vi "Gen Cycle.vi"(7 "Real Time State":T1, 9 "Gen East":T2 {"TotalFuel(L)" format="%.2f"; "FuelRate(L/H)" format="%.2f"; "ApparentPower(VA)" format="%.2f"; "BattVoltage(V)" format="%.2f"; "Freq(Hz)" format="%.2f"; "RunHours(hr)" format="%.2f"; "PowerFactor" format="%.2f"; "ReactivePower(VAR)" format="%.2f"; "ActivePower(W)" format="%.2f"}, 10 "Gen West":T2 {"TotalFuel(L)" format="%.2f"; "FuelRate(L/H)" format="%.2f"; "ApparentPower(VA)" format="%.2f"; "BattVoltage(V)" format="%.2f"; "Freq(Hz)" format="%.2f"; "RunHours(hr)" format="%.2f"; "PowerFactor" format="%.2f"; "ReactivePower(VAR)" format="%.2f"; "ActivePower(W)" format="%.2f"}, 11 "Generator ON":bool=TRUE) -> (1 "Gen Active":T2 {"TotalFuel(L)" format="%.2f"; "FuelRate(L/H)" format="%.2f"; "ApparentPower(VA)" format="%.2f"; "BattVoltage(V)" format="%.2f"; "Freq(Hz)" format="%.2f"; "RunHours(hr)" format="%.2f"; "PowerFactor" format="%.2f"; "ReactivePower(VAR)" format="%.2f"; "ActivePower(W)" format="%.2f"}, 2 "Generator ON East":bool=TRUE, 3 "Generator ON West":bool=TRUE)   [LabVIEW 2014]
uses:
  Controls/Gen Data.ctl
  Controls/RT State.ctl
panel:
  out "Gen West Not Ready":bool=TRUE
  out "Gen East Not Ready":bool=TRUE
  in  "Hour":i32=12
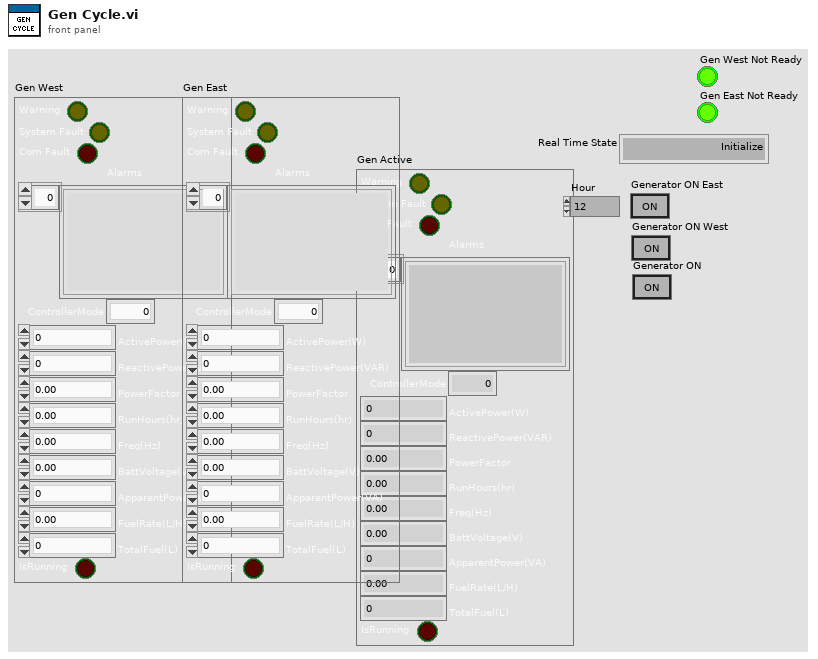
[diagram p1: front panel]
types:
  T1 = typedef "RT State.ctl" = enum16{"Initialize", "Ready", "Startup 1 - Start Genset", "Startup 2 - Start Inverter", "Startup 3 - Battery Match", "SpotGen - Start", "SpotGen - Charge", "SpotGen - Desync", "SpotGen - Discharge", "SpotGen - Sync", "Shutdown", "INVALID STATE"}
  T2 = typedef "Gen Data.ctl" = cluster{"Warning":bool, "System Fault":bool, "Com Fault":bool, "Alarms":string[], "ControllerMode":u16, "ActivePower(W)":i32, "ReactivePower(VAR)":i32, "PowerFactor":dbl, "RunHours(hr)":dbl, "Freq(Hz)":dbl, "BattVoltage(V)":dbl, "ApparentPower(VA)":i32, "FuelRate(L/H)":dbl, "TotalFuel(L)":u32, "IsRunning":bool}
  T3 = typedef "LVDateTimeRec.ctl" = cluster{"fractional second":dbl, "second":i32, "minute":i32, "hour":i32, "day of month":i32, "month":i32, "year":i32, "day of week":i32, "day of year":i32, "DST":i32}
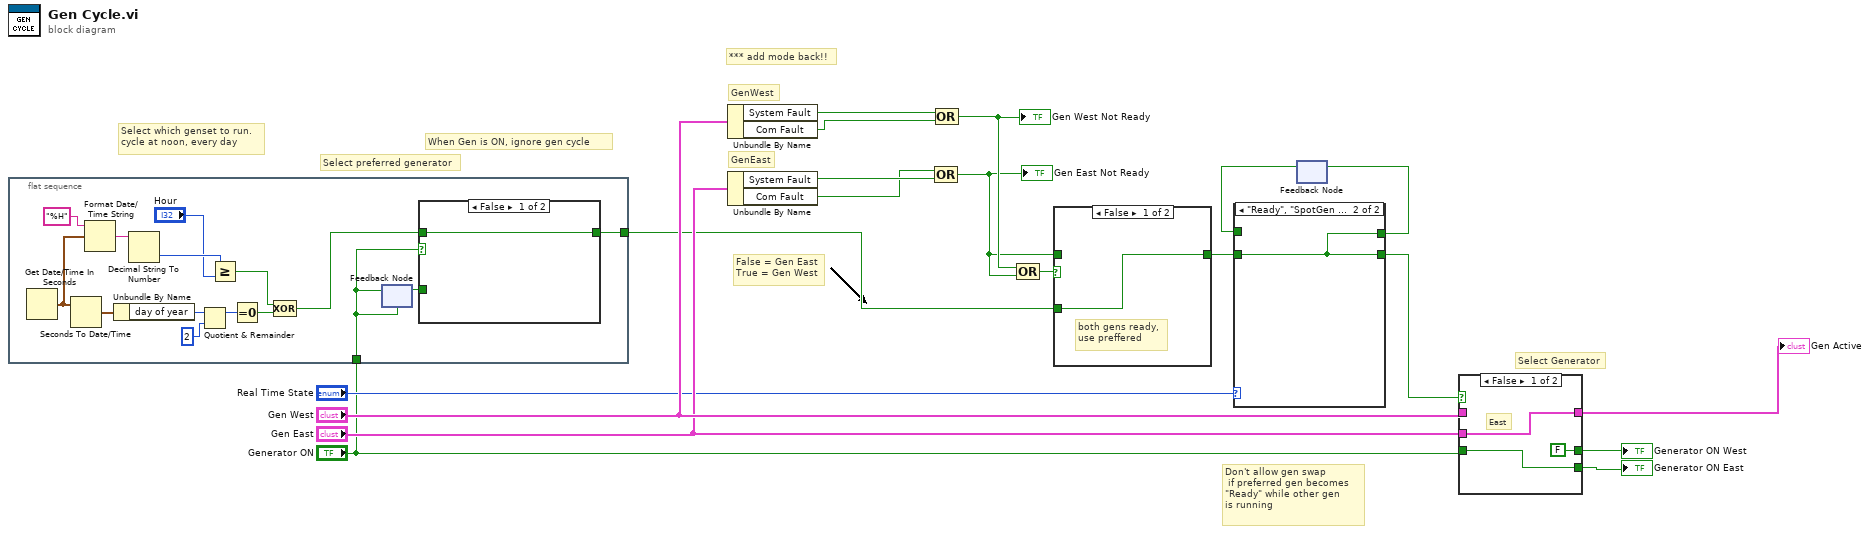
[diagram p0: block diagram]
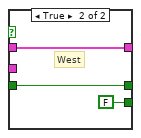
[diagram p4: hidden frame]
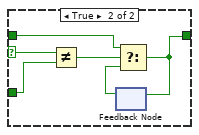
[diagram p5: hidden frame]
diagram:
  # "*** add mode back!!"
  # "GenEast"
  # "GenWest"
  # "Select preferred generator"
  # "Don't allow gen swap \n if preferred gen becomes \n\"Ready\" while other gen \nis running"
  # "Select Generator"
  # "False = Gen East\nTrue = Gen West"
  # "When Gen is ON, ignore gen cycle"
  # "Select which genset to run.\ncycle at noon, every day"
  n1 = flat-sequence {
    tunnel: "Generator ON" -> [w21]
    tunnel: [w20] -> w14
    frame #0 {
      n2 = Get Date/Time In Seconds() -> (seconds since 1Jan1904=w26:timestamp)
      n3 = Seconds To Date/Time(time stamp (now)=w26) -> (date time rec=w34:T3)  [unwired: 1 in]
      n4 = Format Date/Time String(time format string (%c)="%H", seconds (now)=w26) -> (date/time string=w29:string)  [unwired: 1 in]
      n5 = Unbundle By Name(w34) -> ("day of year"=w31:i32)
      n6 = Decimal String To Number(string=w29) -> (number=w28:i32)  [unwired: 2 in, 1 out]
      n7 = Quotient & Remainder(x=w31, y=2) -> (x-y*floor(x/y)=w33:i32)  [unwired: 1 out]
      n8 = Greater Or Equal?(x=w28, y="Hour") -> (x >= y?=w24:bool)
      n9 = Equal To 0?(x=w33) -> (x = 0?=w25:bool)
      n10 = Compound Arithmetic op=XOR(w24, w25) -> (w22:bool)
      n11 = feedback #1(w21) -> (w23:bool)
      n12 = feedback-in #1(w21) -> ()
      n13 = case shown="False" w21 {
        selector: w21 -> [_ w41]
        tunnel: w22 -> [w35 w38]
        tunnel: [w35 w36] -> w20
        tunnel: w23 -> [_ w40]
        frame False {
        }
        frame True {
          n14 = Not Equal?(x=w41, y=w40) -> (x != y?=w39:bool)
          n15 = feedback #2() -> (w37:bool)  [unwired: 1 in]
          n16 = Select(t=w38, s=w39, f=w37) -> (s? t:f=w36:bool)
          n17 = feedback-in #2(w36) -> ()
        }
      }
    }
  }
  n18 = Unbundle By Name("Gen West") -> ("System Fault"=w16:bool, "Com Fault"=w5:bool)
  n19 = Unbundle By Name("Gen East") -> ("System Fault"=w15:bool, "Com Fault"=w4:bool)
  n20 = Compound Arithmetic op=OR(w4, w15) -> (w11:bool)
  "Gen East Not Ready" <- w11
  n21 = Compound Arithmetic op=OR(w16, w5) -> (w12:bool)
  "Gen West Not Ready" <- w12
  n22 = Compound Arithmetic op=OR(w12, w11) -> (w13:bool)
  n23 = case shown="False" w13 {
    tunnel: w14 -> [w42 _]
    tunnel: [w42 w43] -> w10
    tunnel: w11 -> [_ w43]
    frame False {
      # "both gens ready,\nuse preffered"
    }
    frame True {
      # "If one gen is not \nready, use the other"
    }
  }
  n24 = feedback #3() -> (w8:bool)  [unwired: 1 in]
  n25 = case shown="\"Ready\", \"SpotGen - Discharge\"..\"Shutdown\"" "Real Time State" {
    tunnel: w10 -> [_ w45]
    tunnel: [w44 w45] -> w7
    tunnel: w8 -> [w44 _]
    tunnel: [w44 w45] -> w6
    frame "Initialize", Default {
    }
    frame "Ready", "SpotGen - Discharge".."Shutdown" {
    }
  }
  n26 = feedback-in #3(w6) -> ()
  n27 = case shown="False" w7 {
    tunnel: "Gen West" -> [_ w49]
    tunnel: "Gen East" -> [w46 _]
    tunnel: "Generator ON" -> [w48 w51]
    tunnel: [w46 w49] -> w19
    tunnel: [FALSE ("Generator ON") w51] -> w2
    tunnel: [w48 FALSE ("Generator ON")] -> w1
    frame False {
      # "East"
    }
    frame True {
      # "West"
    }
  }
  "Generator ON West" <- w2
  "Generator ON East" <- w1
  "Gen Active" <- w19
